vi "Async Get image from CamServer and display locally.vi"(2 "Image name":string="test", 3 "Image directory path":path=path "C:/test", 4 "Camera":T2="Travcam") -> (0 "Error out":errorcluster, 1 "Image file path":path)   [LabVIEW 2015]
doc: "Asynchronously gets a snapshot image from the selected camera on the camera server and saves it to the specified path with specified name. The VI then shows its front panel with the image."
uses:
  Camera enum/Camera enum.ctl
  <vilib>/vision/Image Controls.llb/IMAQ Image.ctl
  Globals/CamServer global.vi
panel:
  out "Image":T1(plugin-control)
  # "PN 21/08/15"
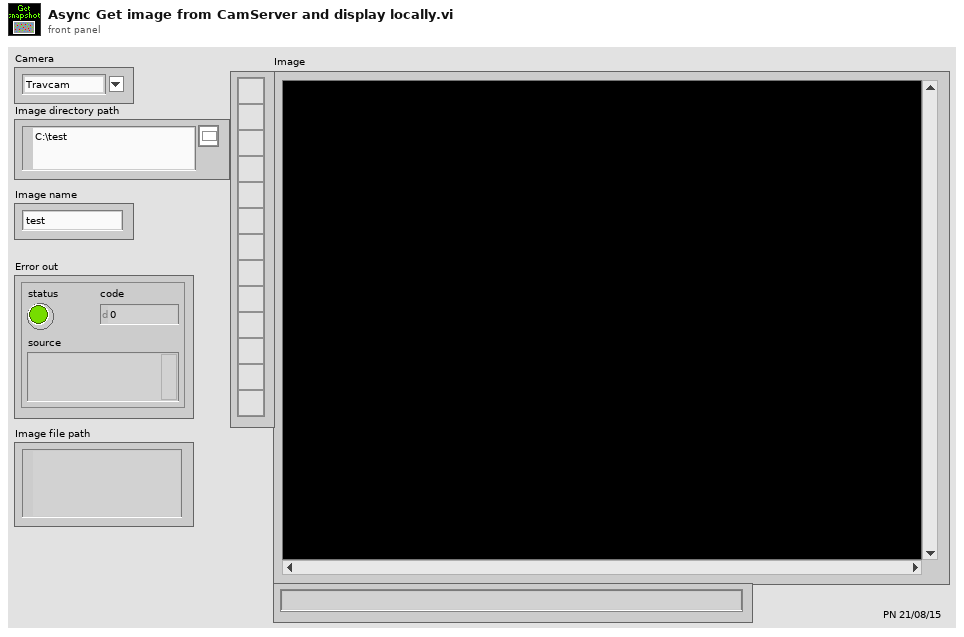
[diagram p1: front panel]
types:
  T1 = typedef "IMAQ Image.ctl" = refnum<image>
  T2 = typedef "Camera enum.ctl" = string
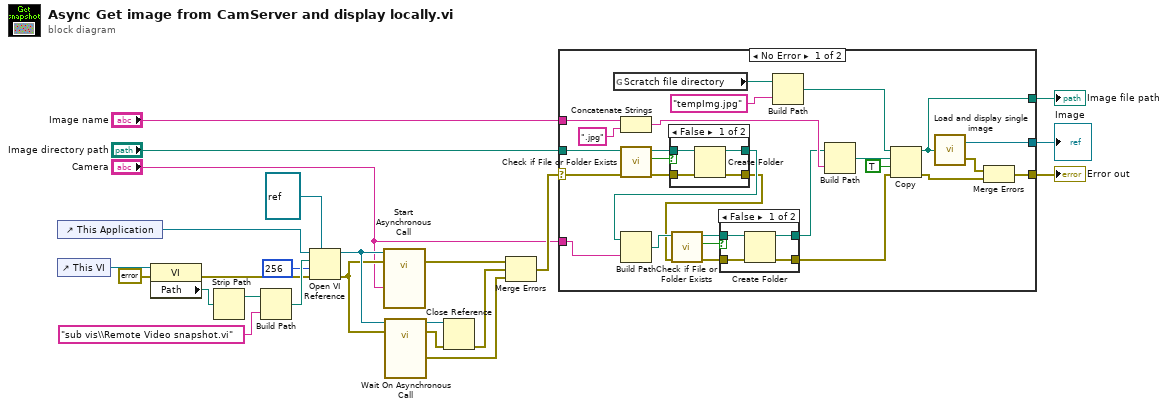
[diagram p0: block diagram]
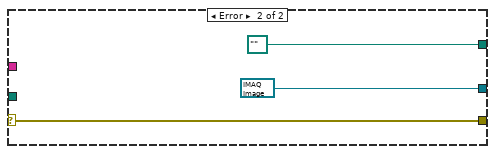
[diagram p4: hidden frame]
diagram:
  n1 = control-ref of="This Application"() -> (w19:refnum<vi>)
  n2 = control-ref of="This VI"() -> (w24:refnum<vi>)
  n3 = property class="VI"(reference=w24, error in=errorcluster {"status"=FALSE, "code"=0, "source"=""} ("error in (no error)")) -> (error out=w21:errorcluster, "Path"=w17:path)  [unwired: 1 out]
  n4 = Strip Path(path=w17) -> (stripped path=w16:path)  [unwired: 1 out]
  n5 = Build Path(base path=w16, name or relative path="sub vis\\Remote Video snapshot.vi") -> (appended path=w22:path)
  n6 = Open VI Reference(type specifier VI Refnum (for type only)=refnum<vi> refnum, application reference (local)=w19, vi path=w22, options=256, error in (no error)=w21) -> (vi reference=w15:refnum<vi>, error out=w14:errorcluster)  [unwired: 1 in]
  n7 = call-by-ref "Start Asynchronous Call"(reference=w15, error in=w14, "Camera"="Camera") -> (error out=w12:errorcluster)  [unwired: 2 out]
  n8 = call-by-ref "Wait On Asynchronous Call"(reference=w15, error in=w14) -> (reference out=w13:refnum<vi>, error out=w11:errorcluster, "Error out"=w9:errorcluster)  [unwired: 1 in]
  n9 = Close Reference(reference=w13, error in (no error)=w11) -> (error out=w10:errorcluster)
  n10 = Merge Errors(w12, w10, w9) -> (w5:errorcluster)
  n11 = case shown="No Error" w5 {
    selector: w5 -> [w50 w66]
    tunnel: "Image directory path" -> [w51 _]
    tunnel: "Image name" -> [w45 _]
    tunnel: [w39 w66] -> w2
    tunnel: [w38 T1 refnum ("Image")] -> w3
    tunnel: "Camera" -> [w30 _]
    tunnel: [w25 path "" ("new path")] -> w1
    frame No Error {
      n12 = global read "CamServer global.vi" "Scratch file directory"() -> (w40:path)
      n13 = Concatenate Strings(w45, ".jpg" ("string")) -> (w43:string)
      n14 = call <vilib>:"Check if File or Folder Exists.vi"("error in (no error)"=w50, "path"=w51) -> ("error out"=w47:errorcluster, "file or folder exists?"=w49:bool, "dup path"=w48:path)  [unwired: 7 in]
      n15 = case shown="False" w49 {
        tunnel: w48 -> [w61 w63]
        tunnel: w47 -> [w60 w62]
        tunnel: [w59 w63] -> w31
        tunnel: [w58 w62] -> w28
        frame False {
          n16 = Create Folder(path (use dialog)=w61, error in=w60) -> (created path=w59:path, error out=w58:errorcluster)  [unwired: 1 in, 1 out]
        }
        frame True {
        }
      }
      n17 = Build Path(base path=w31, name or relative path=w30) -> (appended path=w29:path)
      n18 = call <vilib>:"Check if File or Folder Exists.vi"("error in (no error)"=w28, "path"=w29) -> ("error out"=w32:errorcluster, "file or folder exists?"=w33:bool, "dup path"=w34:path)  [unwired: 7 in]
      n19 = case shown="False" w33 {
        tunnel: w34 -> [w55 w57]
        tunnel: w32 -> [w54 w56]
        tunnel: [w53 w57] -> w27
        tunnel: [w52 w56] -> w26
        frame False {
          n20 = Create Folder(path (use dialog)=w55, error in=w54) -> (created path=w53:path, error out=w52:errorcluster)  [unwired: 1 in, 1 out]
        }
        frame True {
        }
      }
      n21 = Build Path(base path=w40, name or relative path="tempImg.jpg") -> (appended path=w36:path)
      n22 = Build Path(base path=w27, name or relative path=w43) -> (appended path=w44:path)
      n23 = Copy(8:w26, 9:TRUE ("overwrite (F)"), 10:w44, 11:w36) -> (0:w37:errorcluster, 3:w25:path)  [unwired: 1 in, 1 out]
      n24 = call "Load and display single image.vi"("Image file path"=w25) -> ("Image"=w38:T1, "Load image error"=w35:errorcluster)
      n25 = Merge Errors(w35, w37) -> (w39:errorcluster)
    }
    frame Error {
    }
  }
  "Error out" <- w2
  "Image" <- w3
  "Image file path" <- w1
